vi "CreateWaveform.vi"(8 "error in (no error)":errorcluster, 10 "YArrayType":refnum<class "LVType.lvclass">, 11 "ID":string) -> (0 "error out":errorcluster, 3 "LVAnalogWaveformType out":refnum<class "LVAnalogWaveformType.lvclass">)   [LabVIEW 2020, in "LVDataTypes.lvlib" / "LVAnalogWaveformType.lvclass"]
uses:
  <vilib>/AppBuilder/Engine/WebServiceDescription/LVDataTypes/LVAnalogWaveformType/LVAnalogWaveformType.lvclass
  e:/builds/penguin/labview/branches/2020/dev/dist/vi.lib/AppBuilder/Engine/WebServiceDescription/LVDataTypes/LVType/LVType.lvclass
  <vilib>/AppBuilder/Engine/WebServiceDescription/LVDataTypes/LVType/LVType.lvclass
  <vilib>/AppBuilder/Engine/WebServiceDescription/LVDataTypes/TypeCode.ctl
  <vilib>/AppBuilder/Engine/WebServiceDescription/LVDataTypes/LVAnalogWaveformType/LVAnalogWaveformType.lvclass/LVAnalogWaveformType.ctl
  <vilib>/AppBuilder/Engine/WebServiceDescription/LVDataTypes/LVDataTypes.lvlib
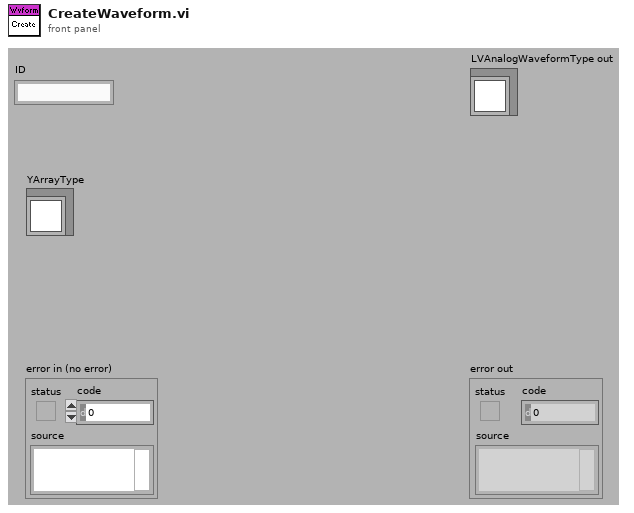
[diagram p1: front panel]
types:
  T1 = typedef "LVDataTypes.lvlib/TypeCode.ctl" = enum16{"Undefined", "Byte", "Unsigned Byte", "Word", "Unsigned Word", "Long", "Unsigned Long", "Quad", "Unsigned Quad", "Single", "Double", "Extended", "Enum", "Boolean", "String", "Path", "Array", "Cluster", "AnalogWaveform", "DigitalWaveform", "Time Stamp", "Void", "Complex Single", "Complex Double", "Complex Extended"}
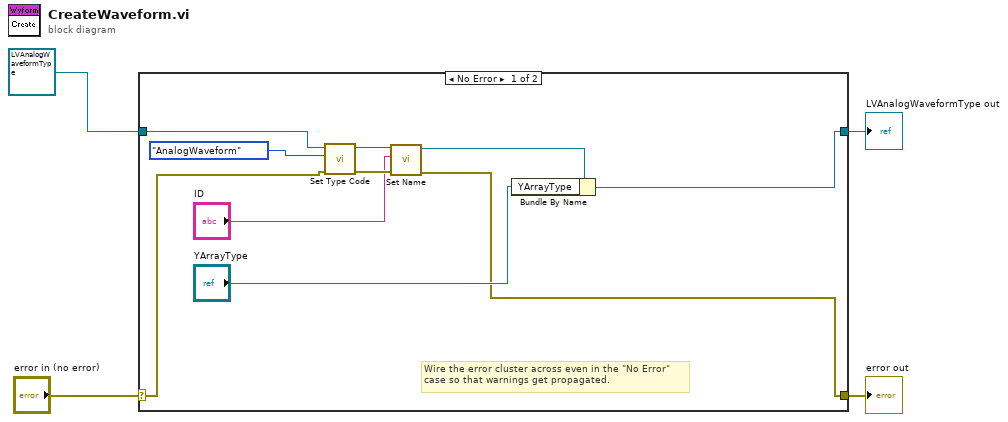
[diagram p0: block diagram]
diagram:
  n1 = case shown="No Error" "error in (no error)" {
    selector: "error in (no error)" -> [w8 w16]
    tunnel: [w6 w16] -> w3
    tunnel: [w13 w15] -> w1
    tunnel: refnum<class "LVAnalogWaveformType.lvclass"> refnum ("LVAnalogWaveformType in") -> [w10 w15]
    frame No Error {
      # "Wire the error cluster across even in the \"No Error\"\ncase so that warnings get propagated."
      n2 = call <vilib>:"Set Type Code.vi"("error in (no error)"=w8, "Type"=TypeCode."AnalogWaveform", "LVType.lvclass in"=w10) -> ("error out"=w11:errorcluster, "LVType.lvclass out"=w12:refnum<class "LVAnalogWaveformType.lvclass">)  [unwired: 7 out]
      n3 = call <vilib>:"Set Name.vi"("error in (no error)"=w11, "Name"="ID", "LVType.lvclass in"=w12) -> ("error out"=w6:errorcluster, "LVType.lvclass out"=w7:refnum<class "LVAnalogWaveformType.lvclass">)  [unwired: 7 out]
      n4 = Bundle By Name(cluster=w7, "YArrayType"="YArrayType") -> (w13:refnum<class "LVAnalogWaveformType.lvclass">)
    }
    frame Error {
    }
  }
  "error out" <- w3
  "LVAnalogWaveformType out" <- w1
